vi "Pre Launch Init.vi"(11 "Nested in":refnum<class "Doña Rata Actor.lvclass">) -> (0 "error out":errorcluster, 3 "Nested out":refnum<class "Doña Rata Actor.lvclass">)   [LabVIEW 2020, in "Doña Rata Actor.lvlib" / "Doña Rata Actor.lvclass"]
doc: "(<B>Filename</B>: Actor Framework.lvlib:Actor.lvclass:Pre Launch Init.vi)\n\nDefines behavior that occurs after the Launch Nested Actor method is invoked but before the actor's Actor Core method begins running.\n\nBy default, this method does nothing. A descendant class may override it to define behavior."
uses:
  <vilib>/ActorFramework/Actor/Actor.lvclass
  C:/Program Files/National Instruments/LabVIEW 2020/vi.lib/ActorFramework/Actor/Actor.lvclass
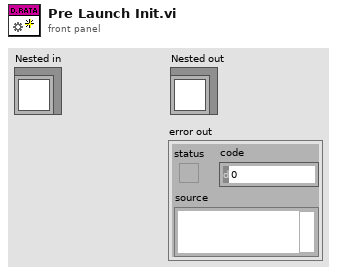
[diagram p1: front panel]
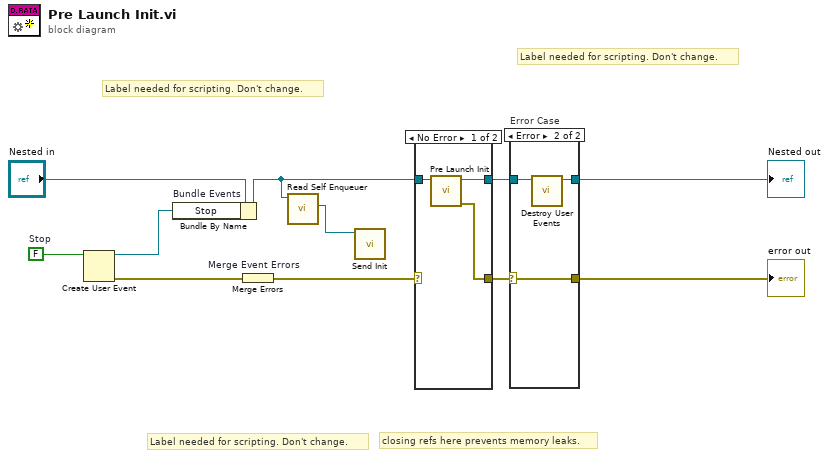
[diagram p0: block diagram]
diagram:
  w10 = FALSE  # Stop
  # "Label needed for scripting. Don't change."
  # "Label needed for scripting. Don't change."
  # "Label needed for scripting. Don't change."
  # "closing refs here prevents memory leaks."
  n1 = Create User Event(user event datatype=w10) -> (user event=w7:refnum<user-event>, error out=w9:errorcluster)  [unwired: 1 in]
  n2 = Bundle By Name "Bundle Events"(cluster="Nested in", "Stop"=w7) -> (w2:refnum<class "Doña Rata Actor.lvclass">)
  n3 = Merge Errors "Merge Event Errors"(w9) -> (w4:errorcluster)
  n4 = call <vilib>:"Read Self Enqueuer.vi"("Actor"=w2) -> ("Self Enqueuer"=w1:refnum<class "Message Enqueuer.lvclass">)  [unwired: 10 in]
  n5 = call "Send Init.vi"("Message Enqueuer"=w1) -> ()  [unwired: 9 in, 2 out]
  n6 = case shown="No Error" w4 {
    selector: w4 -> [_ w16]
    tunnel: [w14 w15] -> w5
    tunnel: w2 -> [w13 w15]
    tunnel: [w12 w16] -> w3
    frame No Error {
      n7 = call-parent "Pre Launch Init.vi"("Actor in"=w13) -> ("error out"=w12:errorcluster, "Actor out"=w14:refnum<class "Doña Rata Actor.lvclass">)  [unwired: 9 in]
    }
    frame Error {
    }
  }
  n8 = case "Error Case" shown="Error" w3 {
    selector: w3 -> [w17 w21]
    tunnel: w5 -> [w18 w20]
    tunnel: [w18 w19] -> w8
    tunnel: [w17 w21] -> w6
    frame No Error {
    }
    frame Error {
      n9 = call "Destroy User Events.vi"("UI Template in"=w20) -> ("UI Template out"=w19:refnum<class "Doña Rata Actor.lvclass">)  [unwired: 10 in]
    }
  }
  "error out" <- w6
  "Nested out" <- w8
